vi "Test 4.vi"(8 "error in (no error)":errorcluster, 11 "Test Case In":refnum<class "Tests.lvclass">) -> (0 "error out":errorcluster, 3 "Test Case Out":refnum<class "Tests.lvclass">)   [LabVIEW 2021, in "Tests.lvclass"]
uses:
  Tests.lvclass
  Tests.lvclass/Tests.ctl
  4993e8ee-a06a-463a-9684-69129f64d5ce.vi
  Proto/Instruction.lvclass
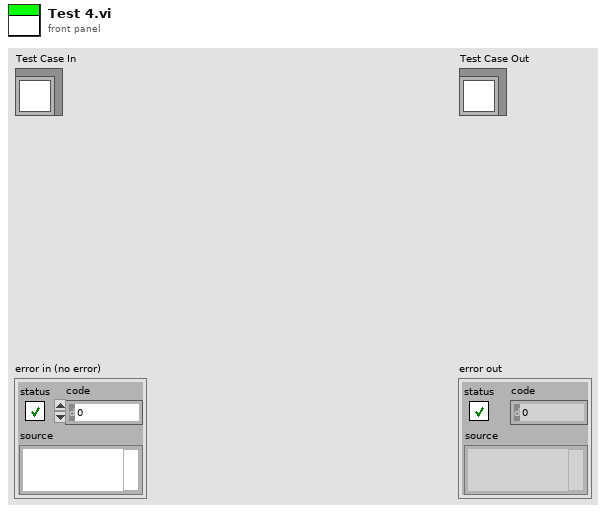
[diagram p1: front panel]
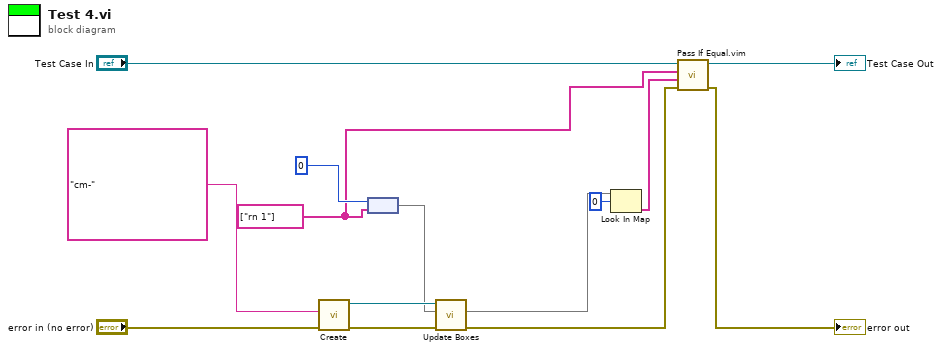
[diagram p0: block diagram]
diagram:
  w1 = string[] ["rn 1"] ("value")
  n1 = call "Create.vi"("error in (no error)"="error in (no error)", "Input"="cm-") -> ("error out"=w10:errorcluster, "Proto"=w8:refnum<class "Instruction.lvclass">)  [unwired: 8 in]
  n2 = node(0 ("dimension size"), w1) -> (w2:map{i32, string[]})
  n3 = call "Update Boxes.vi"("error in (no error)"=w10, "Boxes"=w2, "Instruction In"=w8) -> ("error out"=w9:errorcluster, "Boxes out"=w6:map{i32, string[]})  [unwired: 6 in, 1 out]
  n4 = Look In Map(map=w6, key=0) -> (value=w4:string[])  [unwired: 1 in, 1 out]
  n5 = call "Pass If Equal.vim"("error in (no error)"=w9, "Actual"=w4, "Expected"=w1, "LUnit Test Case In"="Test Case In") -> ("error out"=→"error out":errorcluster, "LUnit Test Case Out"=→"Test Case Out":refnum<class "Tests.lvclass">)  [unwired: 6 in]
